vi "对ROI进行阈值分割.vi"() -> ()   [LabVIEW 2018]
uses:
  <vilib>/vision/NI_Vision_Development_Module.lvlib
panel:
  out "# of Particles found":i32
  in  "Connectivity":bool
  out "Region Reports":T1(array[cluster]) {"Mean Value" format="%.2f"; "%" format="%.2f"; "Area (calibrated)" format="%.2f"; "Maximal Value" format="%.2f"; "Minimal Value" format="%.2f"; "Standard Variation" format="%.2f"}
  out "Labeled":T2(plugin-control)
  in  "Threshold Values":T3(slide)={"Minimum Value"=0.0, "Maximum Value"=65.106384} scale=0.0..255.0
  in  "Stop":bool
  out "Original":T2(plugin-control)
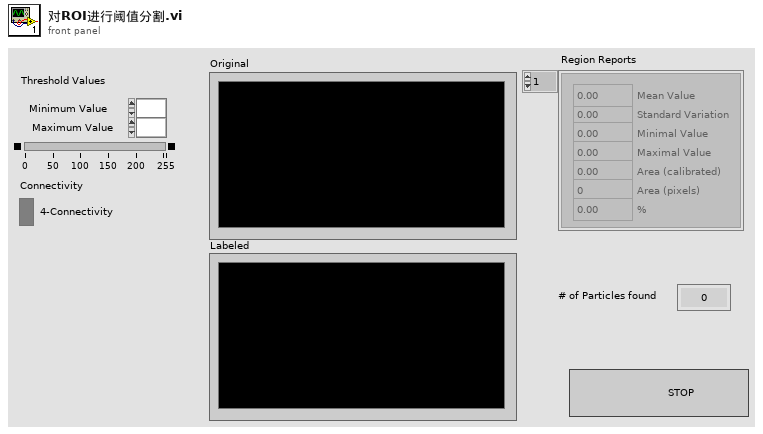
[diagram p1: front panel]
types:
  T1 = cluster{"Mean Value":sgl, "Standard Variation":sgl, "Minimal Value":sgl, "Maximal Value":sgl, "Area (calibrated)":sgl, "Area (pixels)":i32, "%":sgl}[]
  T2 = typedef "IMAQ Image.ctl" = refnum<image>
  T3 = cluster{"Minimum Value":sgl, "Maximum Value":sgl}
  T4 = typedef "Image Type" = u32
  T5 = enum32{"AutoM", "Close", "Dilate", "Erode", "Gradient", "Gradient out", "Gradient in", "Hit miss", "Open", "PClose", "POpen", "Thick", "Thin"}
  T6 = cluster{"Minimum Value":bool, "Maximum Value":bool}
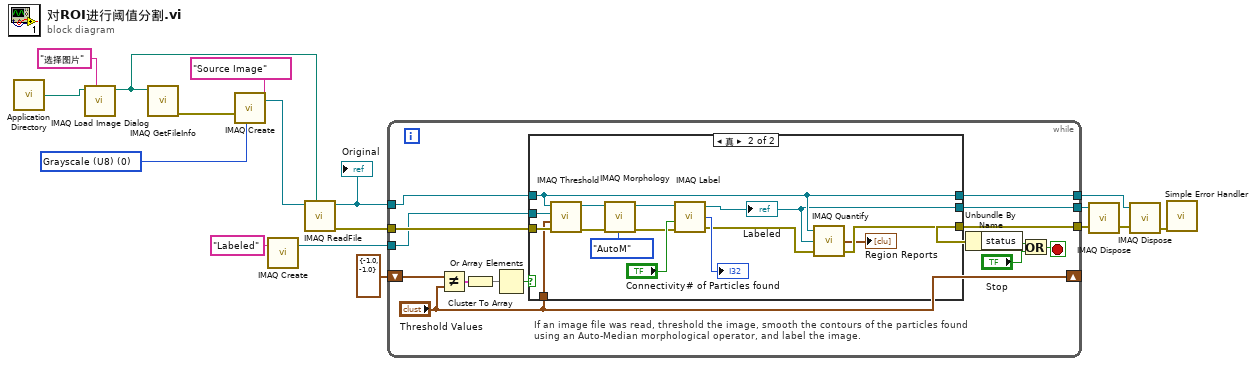
[diagram p0: block diagram]
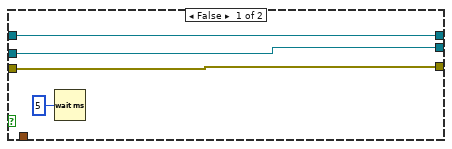
[diagram p2: hidden frame]
diagram:
  w3 = T4 0 items=["Grayscale (U8)", "Grayscale (I16)", "Grayscale (SGL)", "Complex (CSG)", "RGB (U32)", "HSL (U32)", "RGB (U64)", "Grayscale (U16)"] ("Image Type")
  n1 = call <vilib>:"Application Directory.vi"() -> ("Application Directory"=w4:path)
  n2 = call "IMAQ Load Image Dialog"("Prompt"="选择图片" ("prompt"), "Start Path"=w4) -> ("Path"=w2:path)  [unwired: 7 in, 2 out]
  n3 = call "IMAQ GetFileInfo"("File Path"=w2) -> ("error out"=w6:errorcluster)  [unwired: 4 in, 6 out]
  n4 = call "IMAQ Create"("Image Name"="Source Image", "Image Type"=w3, "error in (no error)"=w6) -> ("New Image"=w1:T2)  [unwired: 2 in, 1 out]
  n5 = call "IMAQ Create"("Image Name"="Labeled") -> ("New Image"=w14:T2)  [unwired: 4 in, 1 out]
  n6 = call "IMAQ ReadFile"("File Path"=w2, "Image"=w1) -> ("error out"=w15:errorcluster, "Image Out"=w16:T2)  [unwired: 5 in, 3 out]
  "Original" <- w16
  n7 = while {
    tunnel: w16 -> [w31]
    tunnel: w15 -> [w30]
    tunnel: w14 -> [w29]
    shift-right: ["Threshold Values"] -> _
    shift-left: T3 {"Minimum Value"=-1.0, "Maximum Value"=-1.0} ("Threshold Values") -> [w28]
    tunnel: [w18] -> w9
    tunnel: [w19] -> w11
    tunnel: [w20] -> w12
    stop <- w22 stop-if-true
    # "If an image file was read, threshold the image, smooth the contours of the particles found using an Auto-Median morphological operator, and label the image."
    n8 = Not Equal?(x=w28, y="Threshold Values") -> (x != y?=w27:T6)
    n9 = Cluster To Array(cluster=w27) -> (array=w26:bool[])
    n10 = Or Array Elements(Boolean array=w26) -> (logical OR=w25:bool)
    n11 = case shown="真" w25 {
      tunnel: w31 -> [w32 w38]
      tunnel: w30 -> [w34 w45]
      tunnel: w29 -> [w33 w44]
      tunnel: "Threshold Values" -> [_ w41]
      tunnel: [w34 w39] -> w20
      tunnel: [w33 w36] -> w19
      tunnel: [w32 w38] -> w18
      frame False {
        n12 = Wait (ms)(milliseconds to wait=u32 5) -> ()  [unwired: 1 out]
      }
      frame True {
        n13 = call "IMAQ Threshold"("error in (no error)"=w45, "Range"=w41, "Image Dst"=w44, "Image Src"=w38) -> ("error out"=w43:errorcluster, "Image Dst Out"=w49:T2)  [unwired: 6 in]
        n14 = call "IMAQ Morphology"("error in (no error)"=w43, "Operation"=T5."AutoM", "Image Src"=w49) -> ("error out"=w42:errorcluster, "Image Dst Out"=w46:T2)  [unwired: 7 in]
        n15 = call "IMAQ Label"("error in (no error)"=w42, "Connectivity 4/8 (8)"="Connectivity", "Image Src"=w46) -> ("error out"=w40:errorcluster, "Number of Particles"=→"# of Particles found":i32, "Image Dst Out"=w36:T2)  [unwired: 1 in]
        "Labeled" <- w36
        n16 = call "IMAQ Quantify"("error in (no error)"=w40, "Image Mask"=w36, "Image"=w38) -> ("error out"=w39:errorcluster, "Region Reports"=→"Region Reports":T1)  [unwired: 1 out]
      }
    }
    n17 = Unbundle By Name(w20) -> ("status"=w24:bool)
    n18 = Or(x=w24, y="Stop") -> (x .or. y?=w22:bool)
  }
  n19 = call "IMAQ Dispose"("Image"=w11, "error in (no error)"=w12) -> ("error out"=w10:errorcluster)  [unwired: 4 in]
  n20 = call "IMAQ Dispose"("Image"=w9, "error in (no error)"=w10) -> ("error out"=w8:errorcluster)  [unwired: 4 in]
  n21 = call <vilib>:"Simple Error Handler.vi"("error in (no error)"=w8) -> ()  [unwired: 4 in, 5 out]
